vi "Load E-series.vi"(6 "error in (no error)":errorcluster, 9 "INI File":string) -> (0 "error out":errorcluster, 3 "Data Series":T1)   [LabVIEW 2018, in "CSV Series Read.lvlib"]
uses:
  CSV Series Read.lvlib
  Data Series.ctl
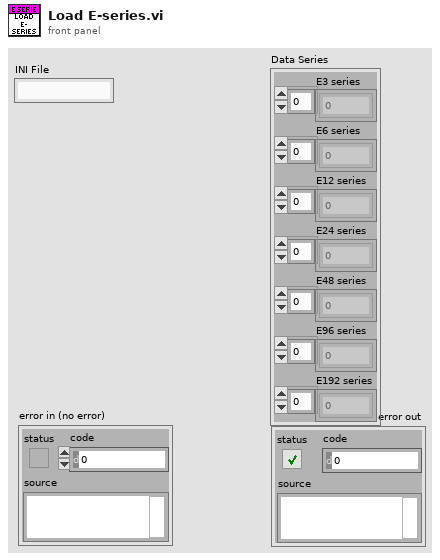
[diagram p1: front panel]
types:
  T1 = typedef "CSV Series Read.lvlib/Data Series.ctl" = cluster{"E3 series":u16[], "E6 series":u16[], "E12 series":u16[], "E24 series":u16[], "E48 series":u16[], "E96 series":u16[], "E192 series":u16[]}
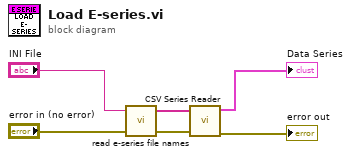
[diagram p0: block diagram]
diagram:
  n1 = call "read e-series file names.vi"("error in (no error)"="error in (no error)", "INI File"="INI File") -> ("error out"=w5:errorcluster, "E-Series File Names"=w6:string[])  [unwired: 2 in]
  n2 = call "CSV Series Reader.vi"("error in"=w5, "Filenames"=w6) -> ("error out"=→"error out":errorcluster, "Data Series"=→"Data Series":T1)  [unwired: 8 in]
